vi "PicoScopeospaNextBuffer.vi"(0 "handle in":i16=16384, 2 "Buffer and Transfer Settings":T3={"startIndex"=0, "Samples"=1000000, "Down Sample Ratio"=1, "Down-Sample Mode"=2147483648} {"Down-Sample Mode" items=["RAW none"=2147483648, "None"=0, "Aggregate"=1, "Decimate"=2, "Average"=4]; "Down Sample Ratio" step=1; "Samples" format="%_6p"}, 3 "enabled array":i16[](array[numeric])=[1, 1, 0, 0, 0, 0, 0, 0, 0, 0], 5 "Device Info":T1, 7 "Data Pointers In":T2, 9 "Buffer Number":i32=1, 11 "error in (no error)":errorcluster, 13 "LoopFlag":bool) -> (4 "handle out":i16=16384, 15 "error out":errorcluster)   [LabVIEW 2010]
doc: "Call GetValues to fill the next set of channel buffers."
uses:
  psospa.dll
  shared/PicoBuffers.ctl
  shared/Buffer and Transfer Settings.ctl
panel:
  in  "SetDataBuffer0 flag":bool
  # "Samples can be equal to or less\nTotal Pre and Post Trigger Samples"
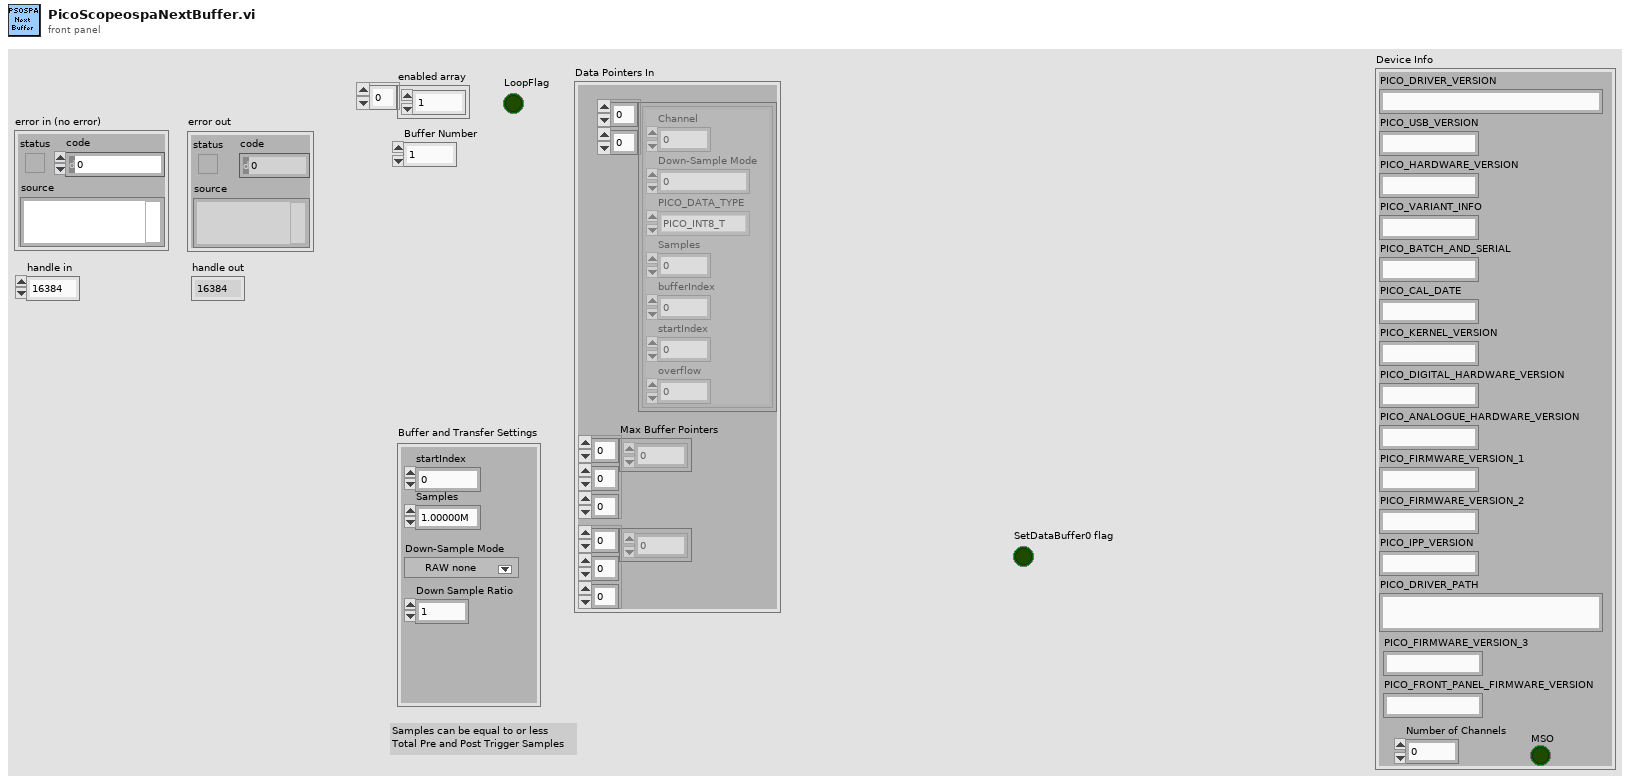
[diagram p1: front panel]
types:
  T1 = cluster{"PICO_DRIVER_VERSION":string, "PICO_USB_VERSION":string, "PICO_HARDWARE_VERSION":string, "PICO_VARIANT_INFO":string, "PICO_BATCH_AND_SERIAL":string, "PICO_CAL_DATE":string, "PICO_KERNEL_VERSION":string, "PICO_DIGITAL_HARDWARE_VERSION":string, "PICO_ANALOGUE_HARDWARE_VERSION":string, "PICO_FIRMWARE_VERSION_1":string, "PICO_FIRMWARE_VERSION_2":string, "PICO_IPP_VERSION":string, "PICO_DRIVER_PATH":string, "PICO_FIRMWARE_VERSION_3":string, "PICO_FRONT_PANEL_FIRMWARE_VERSION":string, "Number of Channels":i16, "MSO":bool}
  T2 = typedef "PicoBuffers.ctl" = cluster{"Max Buffer Pointers":u64[][][], "Min Buffer Pointers":u64[][][], "StreamingDataInfo":cluster{"Channel":u32, "Down-Sample Mode":u32, "PICO_DATA_TYPE":enum32{"PICO_INT8_T", "PICO_INT16_T", "PICO_INT32_T", "PICO_UINT32_T", "PICO_INT64_T", ""}, "Samples":i32, "bufferIndex":u64, "startIndex":i32, "overflow":i16}[][]}
  T3 = typedef "Buffer and Transfer Settings.ctl" = cluster{"startIndex":u64, "Samples":u64, "Down Sample Ratio":u64, "Down-Sample Mode":u32}
  T4 = enum32{"PICO_INT8_T", "PICO_INT16_T", "PICO_INT32_T", "PICO_UINT32_T", "PICO_INT64_T", ""}
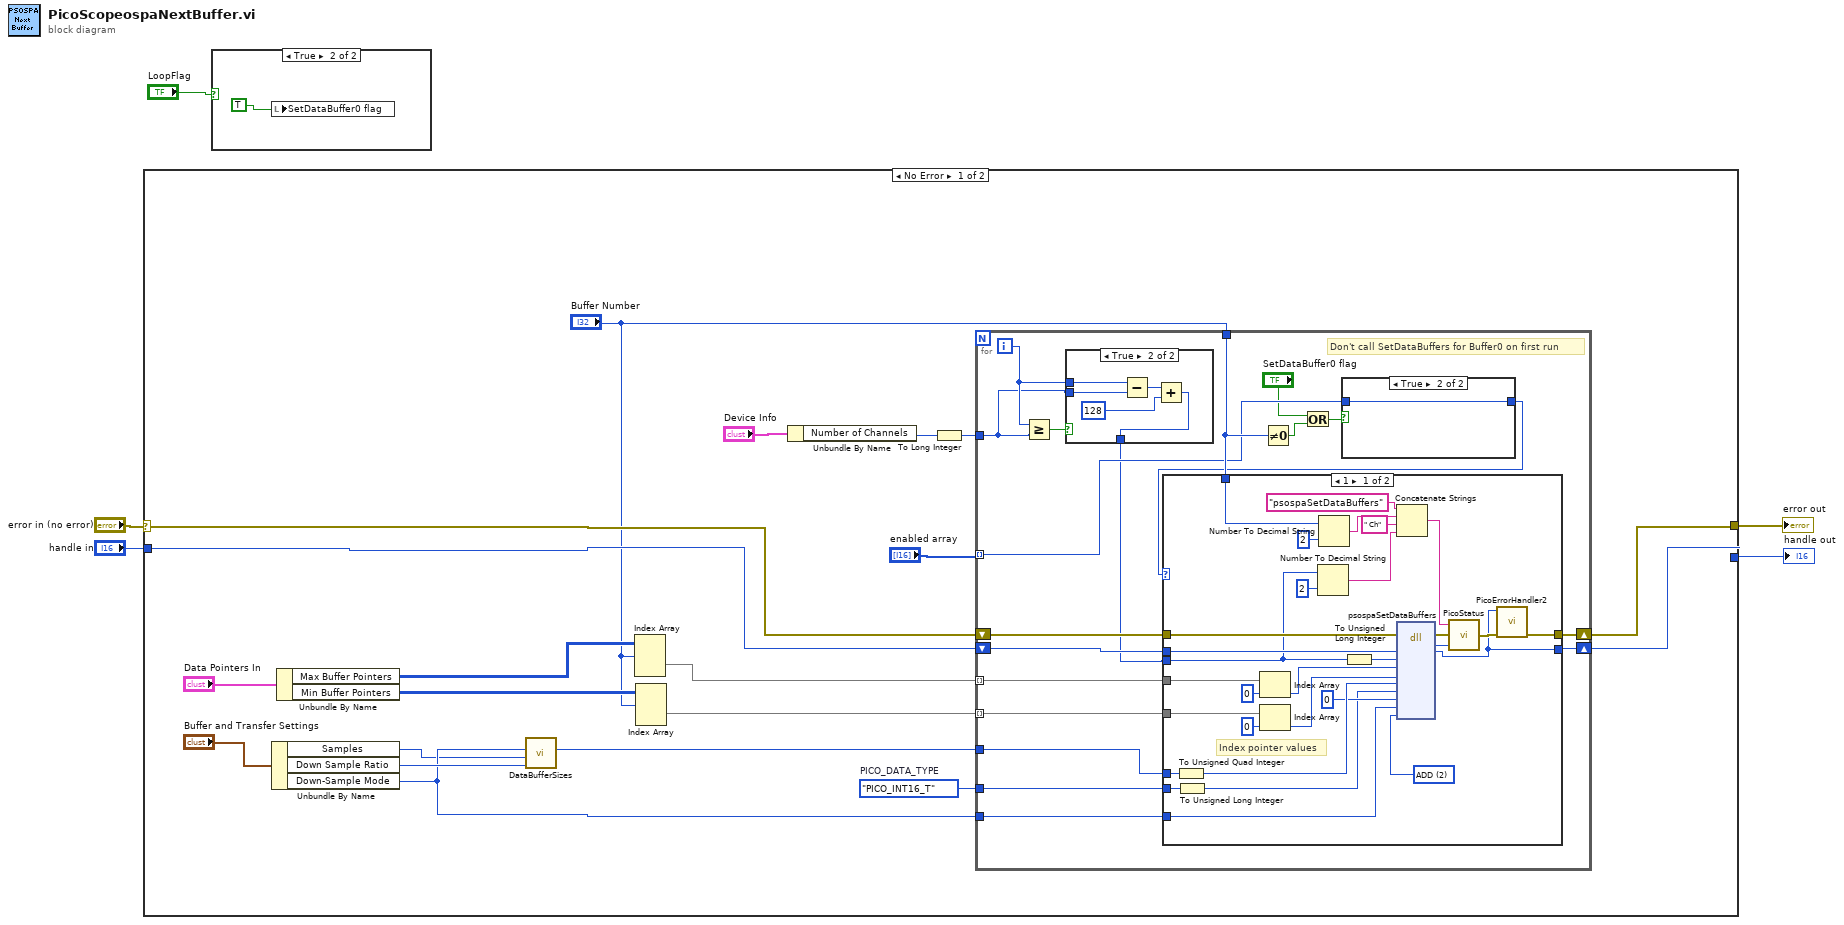
[diagram p0: block diagram]
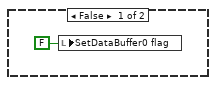
[diagram p2: hidden frame]
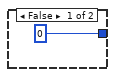
[diagram p4: hidden frame]
diagram:
  n1 = case shown="No Error" "error in (no error)" {
    selector: "error in (no error)" -> [w23 w85]
    tunnel: "handle in" -> [w22 w86]
    tunnel: [w25 w86] -> w3
    tunnel: [w24 w85] -> w2
    frame No Error {
      w7 = T4."PICO_INT16_T"  # PICO_DATA_TYPE
      n2 = Unbundle By Name("Buffer and Transfer Settings") -> ("Samples"=w17:u64, "Down Sample Ratio"=w21:u64, "Down-Sample Mode"=w18:u32)
      n3 = Unbundle By Name("Data Pointers In") -> ("Max Buffer Pointers"=w16:u64[][][], "Min Buffer Pointers"=w15:u64[][][])
      n4 = call "DataBufferSizes.vi"("Down Sample Ratio"=w21, "Number of Samples"=w17, "Down-Sample Mode"=w18) -> ("Max Buffer Size"=w19:i32)  [unwired: 7 in, 1 out]
      n5 = Index Array(array=w16, index (dim 0)="Buffer Number") -> (element=w8:u64[][])  [unwired: 2 in]
      n6 = Index Array(array=w15, index (dim 0)="Buffer Number") -> (element=w9:u64[][])  [unwired: 2 in]
      n7 = Unbundle By Name("Device Info") -> ("Number of Channels"=w12:i16)
      n8 = To Long Integer(number=w12) -> (32bit integer=w10:i32)
      n9 = for {
        tunnel: w18 -> [w44]
        tunnel: w7 -> [w43]
        tunnel: w19 -> [w40]
        tunnel: "enabled array" -> [w36] mode=indexing
        tunnel: "Buffer Number" -> [w39]
        shift-right: [w38] -> w24
        shift-left: w23 -> [w42]
        shift-right: [w37] -> w25
        shift-left: w22 -> [w41]
        tunnel: w8 -> [w31] mode=indexing
        tunnel: w9 -> [w30] mode=indexing
        tunnel: w10 -> [w26]
        i -> [w27]
        # "Don't call SetDataBuffers for Buffer0 on first run"
        n10 = Greater Or Equal?(x=w27, y=w26) -> (x >= y?=w29:bool)
        n11 = case shown="True" w29 {
          tunnel: [w45 w49] -> w28
          tunnel: w26 -> [_ w48]
          tunnel: w27 -> [w45 w47]
          frame False {
          }
          frame True {
            n12 = Subtract(x=w47, y=w48) -> (x-y=w46:i32)
            n13 = Add(x=w46, y=128) -> (x+y=w49:i32)
          }
        }
        n14 = Not Equal To 0?(x=w39) -> (x != 0?=w34:bool)
        n15 = Or(x="SetDataBuffer0 flag", y=w34) -> (x .or. y?=w32:bool)
        n16 = case shown="True" w32 {
          tunnel: [i16 0 ("element") w52] -> w35
          tunnel: w36 -> [_ w52]
          frame False {
          }
          frame True {
          }
        }
        n17 = case shown="1" w35 {
          tunnel: w28 -> [w61 _]
          tunnel: w42 -> [w82 w84]
          tunnel: w41 -> [w79 w83]
          tunnel: w44 -> [w77 _]
          tunnel: w43 -> [w55 _]
          tunnel: w40 -> [w76 _]
          tunnel: w31 -> [w60 _]
          tunnel: [w74 w84] -> w38
          tunnel: w39 -> [w69 _]
          tunnel: [w65 w83] -> w37
          tunnel: w30 -> [w53 _]
          frame 1 {
            w59 = u32 2 items=["NONE"=0, "CLEAR_ALL"=1, "ADD"=2, "CLEAR_THIS_DATA_BUFFER"=4096, "CLEAR_WAVEFORM_DATA_BUFFERS"=8192, "CLEAR_WAVEFORM_READ_DATA_BUFFERS"=16384] ("PicoAction 3")
            # "Index pointer values"
            n18 = To Unsigned Quad Integer(1:w76) -> (0:w75:u64)
            n19 = To Unsigned Long Integer(number=w55) -> (unsigned 32bit integer=w54:u32)
            n20 = Index Array(array=w60, index=0) -> (element=w63:u64)
            n21 = Index Array(array=w53, index=0) -> (element=w56:u64)
            n22 = Number To Decimal String(number=w61, width (-)=i16 2) -> (decimal integer string=w66:string)
            n23 = Number To Decimal String(number=w69, width (-)=i16 2) -> (decimal integer string=w71:string)
            n24 = To Unsigned Long Integer(number=w61) -> (unsigned 32bit integer=w62:u32)
            n25 = Concatenate Strings("psospaSetDataBuffers" ("source"), w71, " Ch" ("string"), w66) -> (w72:string)
            n26 = dll-call lib="psospa.dll" fn="psospaSetDataBuffers" ("ps3000.dll:_ps3000_open_unit@0")(error in=w82, "handle"=w79, "channel"=w62, "bufferMax"=w63, "bufferMin"=w56, "nSamples"=w75, "dataType"=w54, "waveform"=u64 0, "downSampleRatioMode"=w77, "action"=w59) -> (error out=w81:errorcluster, "PICO_STATUS"=w80:u32, "handle"=w65:i16)  [unwired: 10 in, 1 out]
            n27 = call "PicoStatus.vi"("PICO STATUS"=w80, "error in"=w81, "source"=w72) -> ("error out"=w78:errorcluster)
            n28 = call "PicoErrorHandler2.vi"("error in (no error)"=w78, "handle In"=w65) -> ("error out"=w74:errorcluster)  [unwired: 9 in]
          }
          frame 0, Default {
          }
        }
      }
    }
    frame Error {
    }
  }
  "handle out" <- w3
  "error out" <- w2
  n29 = case shown="True" "LoopFlag" {
    frame False {
      n30 = local write "SetDataBuffer0 flag"(FALSE ("SetDataBuffer0 flag")) -> ()
    }
    frame True {
      n31 = local write "SetDataBuffer0 flag"(TRUE ("SetDataBuffer0 flag")) -> ()
    }
  }
